vi "TestArraytoWave.vi"(8 "error in (no error)":errorcluster) -> (0 "error out":errorcluster)   [LabVIEW 2019]
uses:
  lvsrc/private/Igor_NumericArraytoIgorWave.vi
  <vilib>/addons/_JKI Toolkits/Caraya/classes/Assert/Assert Equal Value and Type_Variant.vi
  lvsrc/private/Igor_StringArraytoIgorWave.vi
  <vilib>/addons/_JKI Toolkits/Caraya/classes/Test/Test.lvclass
  <vilib>/addons/_JKI Toolkits/Caraya/classes/Assert/Assert.lvclass
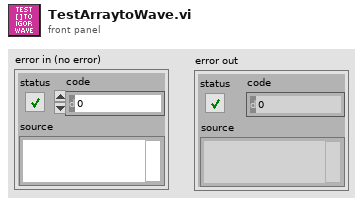
[diagram p1: front panel]
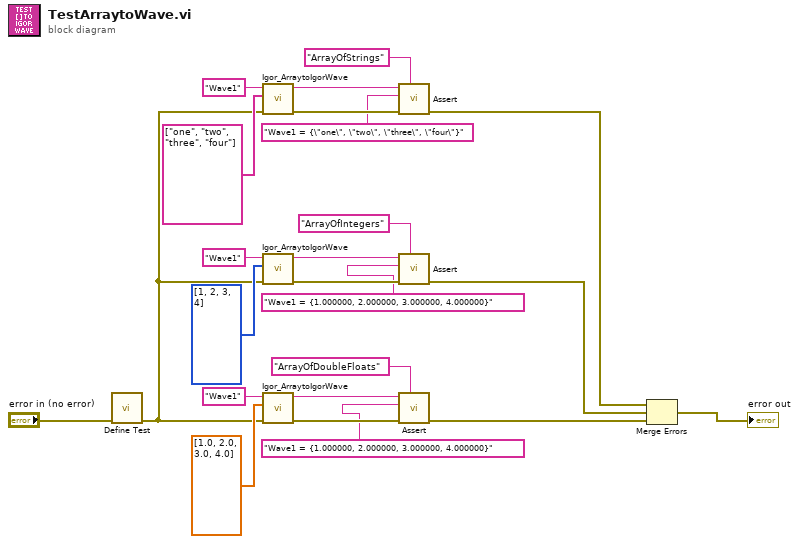
[diagram p0: block diagram]
diagram:
  n1 = call <vilib>:"Define Test.vi"("error in (no error)"="error in (no error)") -> ("error out"=w4:errorcluster)  [unwired: 9 in, 1 out]
  n2 = call-poly "Igor_ArraytoIgorWave.vi"("error in (no error)"=w4, "Wave"=string[] ["one", "two", "three", "four"], "Name"="Wave1") -> ("error out"=w9:errorcluster, "Igor Wave"=w8:string)  [unwired: 7 in]
  n3 = call-poly "Igor_ArraytoIgorWave.vi"("error in (no error)"=w4, "Wave"=i32[] [1, 2, 3, 4], "Name"="Wave1") -> ("error out"=w13:errorcluster, "Igor Wave"=w14:string)  [unwired: 7 in]
  n4 = call-poly "Igor_ArraytoIgorWave.vi"("error in (no error)"=w4, "Wave"=dbl[] [1.0, 2.0, 3.0, 4.0], "Name"="Wave1") -> ("error out"=w20:errorcluster, "Igor Wave"=w19:string)  [unwired: 7 in]
  n5 = call-poly <vilib>:"Assert.vi"("Label"="ArrayOfStrings", "error in (no error)"=w9, "Y"="Wave1 = {\"one\", \"two\", \"three\", \"four\"}", "X"=w8) -> ("error out"=w5:errorcluster)  [unwired: 6 in, 1 out]
  n6 = call-poly <vilib>:"Assert.vi"("Label"="ArrayOfIntegers", "error in (no error)"=w13, "Y"="Wave1 = {1.000000, 2.000000, 3.000000, 4.000000}", "X"=w14) -> ("error out"=w11:errorcluster)  [unwired: 6 in, 1 out]
  n7 = call-poly <vilib>:"Assert.vi"("Label"="ArrayOfDoubleFloats", "error in (no error)"=w20, "Y"="Wave1 = {1.000000, 2.000000, 3.000000, 4.000000}", "X"=w19) -> ("error out"=w22:errorcluster)  [unwired: 6 in, 1 out]
  n8 = Merge Errors(w5, w11, w22) -> (→"error out":errorcluster)
